vi "Stop Move piezo.vi"(8 "error in (no error)":errorcluster, 9 "notifier out":refnum<notifier>, 10 "MOVE TO [MICRON]":dbl=1.0 format="%0.2f", 11 "Cluster":T1={"physical channels"="Dev5/ao0", "MAX   VOLTAGE"=10.0, "MIN   VOLTAGE"=0.0}) -> (0 "error out":errorcluster, 3 "Cluster 2":T1={"physical channels"="Dev5/ao0", "MAX   VOLTAGE"=10.0, "MIN   VOLTAGE"=0.0})   [LabVIEW 2013, in "Piezo.lvlib"]
uses:
  Piezo/Piezo.lvlib
  Piezo/Piezo display.ctl
  Untitled Project 3 Andrea/piezo new/Hardware Configuration Piezo out.ctl
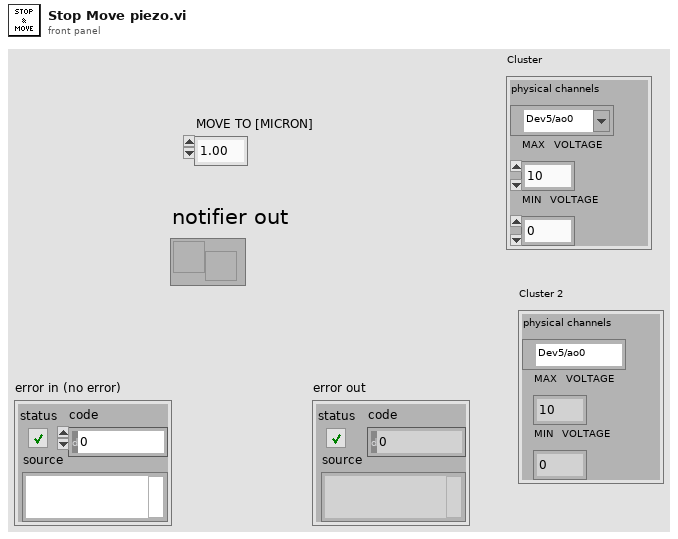
[diagram p1: front panel]
types:
  T1 = typedef "Hardware Configuration Piezo out.ctl" = cluster{"physical channels":tag, "MAX   VOLTAGE":dbl, "MIN   VOLTAGE":dbl}
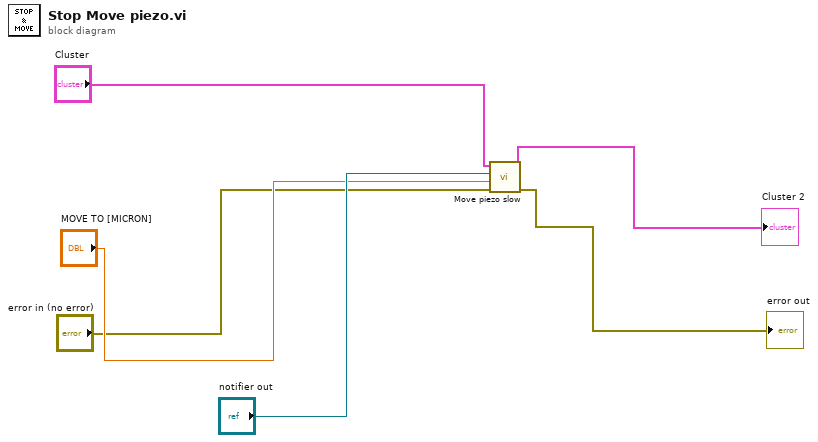
[diagram p0: block diagram]
diagram:
  n1 = call "Move piezo slow.vi"("error in (no error)"="error in (no error)", "MOVE TO [MICRON]"="MOVE TO [MICRON]", "notifier out"="notifier out", "Cluster"="Cluster") -> ("error out"=→"error out":errorcluster, "Cluster 2"=→"Cluster 2":T1)  [unwired: 5 in]
